vi "LAUDA_SEQ.vi"(0 "Numeric 2":dbl, 1 "Numeric 1":dbl, 2 "Numeric":dbl, 5 "Numeric 5":dbl, 7 "Numeric 6":dbl, 9 "Numeric 7":dbl, 12 "Numeric 8":dbl, 13 "Numeric 3":dbl, 14 "Numeric 4":dbl) -> (4 "output array":dbl[](array[numeric]), 6 "output array 2":dbl[](array[numeric]))   [LabVIEW 2015]
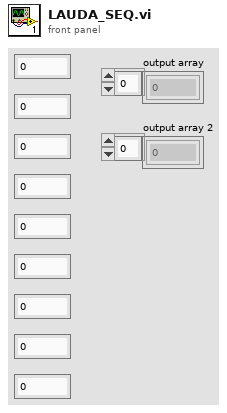
[diagram p1: front panel]
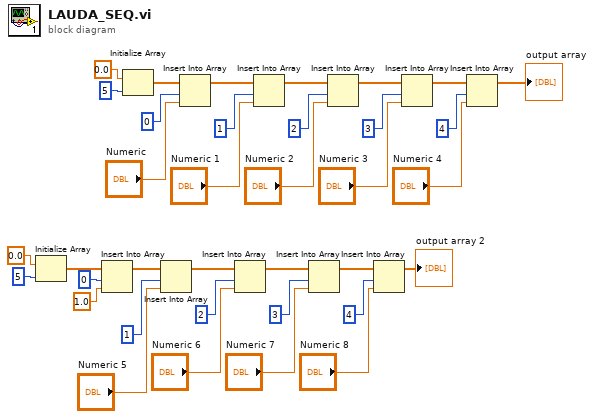
[diagram p0: block diagram]
diagram:
  n1 = Initialize Array(0.0 ("element"), 5 ("dimension size")) -> (w2:dbl[])
  n2 = Insert Into Array(array=w2, index=0, new element=1.0 ("new element/subarray")) -> (w1:dbl[])
  n3 = Initialize Array(0.0 ("element"), 5 ("dimension size")) -> (w7:dbl[])
  n4 = Insert Into Array(array=w1, index=1, new element="Numeric 5") -> (w27:dbl[])
  n5 = Insert Into Array(array=w7, index=0, new element="Numeric") -> (w11:dbl[])
  n6 = Insert Into Array(array=w27, index=2, new element="Numeric 6") -> (w30:dbl[])
  n7 = Insert Into Array(array=w11, index=1, new element="Numeric 1") -> (w14:dbl[])
  n8 = Insert Into Array(array=w30, index=3, new element="Numeric 7") -> (w33:dbl[])
  n9 = Insert Into Array(array=w14, index=2, new element="Numeric 2") -> (w17:dbl[])
  n10 = Insert Into Array(array=w33, index=4, new element="Numeric 8") -> (→"output array 2":dbl[])
  n11 = Insert Into Array(array=w17, index=3, new element="Numeric 3") -> (w20:dbl[])
  n12 = Insert Into Array(array=w20, index=4, new element="Numeric 4") -> (→"output array":dbl[])
